vi "calculate.vi"(9 "专项附加扣除（元）":dbl format="%#.3f", 10 "五险一金扣除（元）":dbl format="%#.3f", 11 "年薪金所得（元）":dbl format="%#.3f") -> (0 "抵扣2":dbl, 1 "抵扣1":dbl, 3 "汇算结果（供参考）":string, 4 "税":dbl, 5 "总收入":dbl)   [LabVIEW 2016, in "Tax_calculation.lvclass"]
uses:
  Tax_calculation.lvclass
  <vilib>/Utility/miscctls.llb/LVPointTypeDef.ctl
  PublicSubvi/BoolACT.ctl
  tax list.vi
panel:
  out "reference out":refnum<vi>
  in  "Tab Control":enum32{"综合年度个税汇算", "月度个税计算（预算）"}(tab)
  in  "list":bool
  in  "RESET":bool
  in  "OK":bool
  # "收入"
  # "扣除"
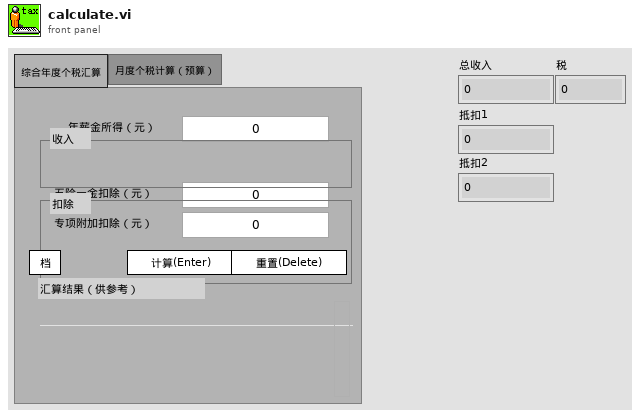
[diagram p1: front panel]
types:
  T1 = typedef "LVPointTypeDef.ctl" = cluster{"Horizontal":i16, "Vertical":i16}
  T2 = cluster{"年薪金所得（元）":refnum<vi>, "五险一金扣除（元）":refnum<vi>, "专项附加扣除（元）":refnum<vi>}
  T3 = enum8{"Enabled", "Disabled", "Disabled and Grayed Out"}
  T4 = typedef "BoolACT.ctl" = enum16{"Get", "Set"}
  T5 = enum32{"Invalid", "Standard", "Closed", "Hidden", "Minimized", "Maximized"}
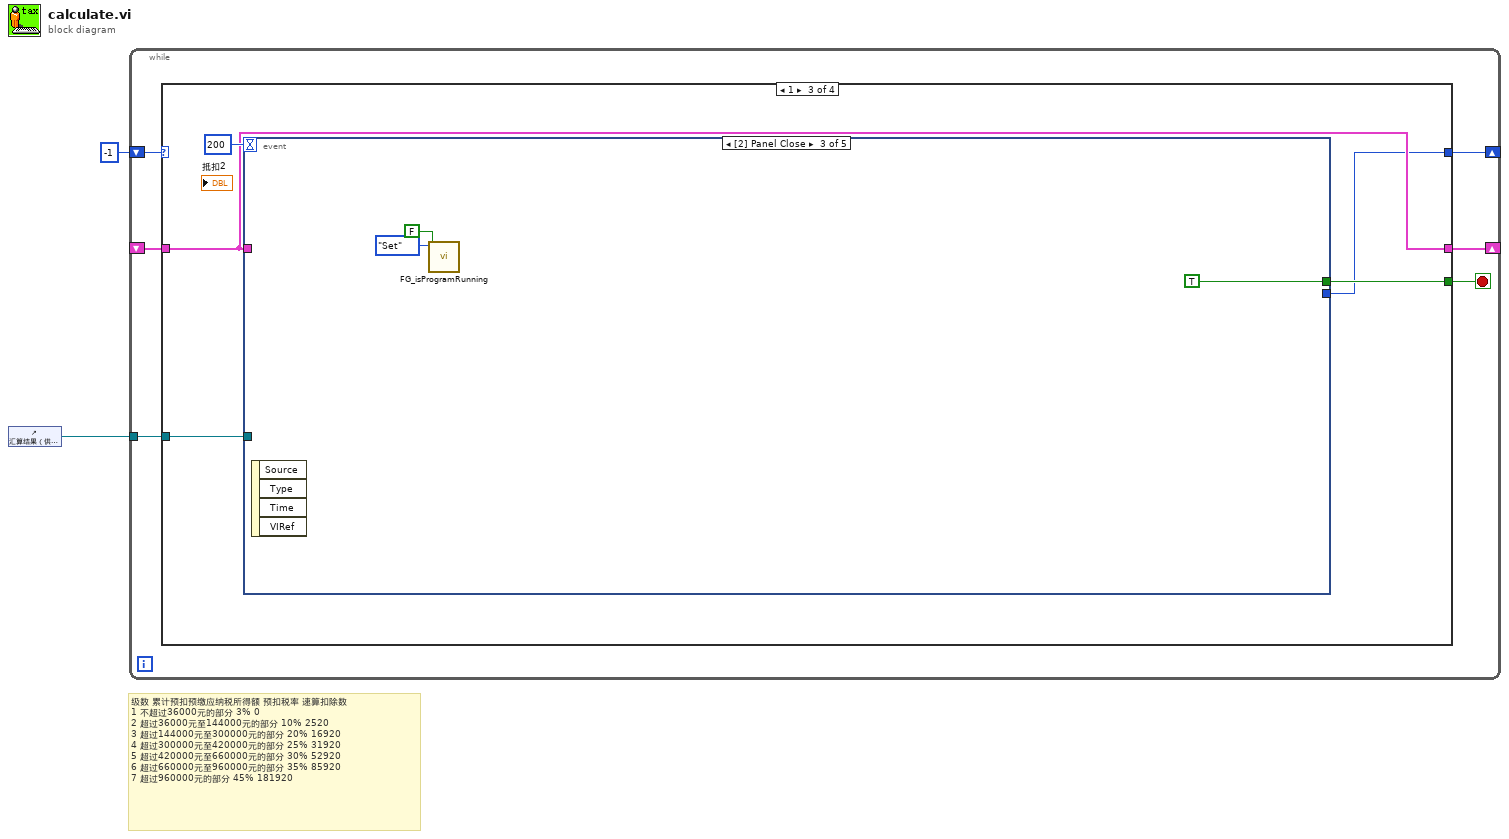
[diagram p0: block diagram]
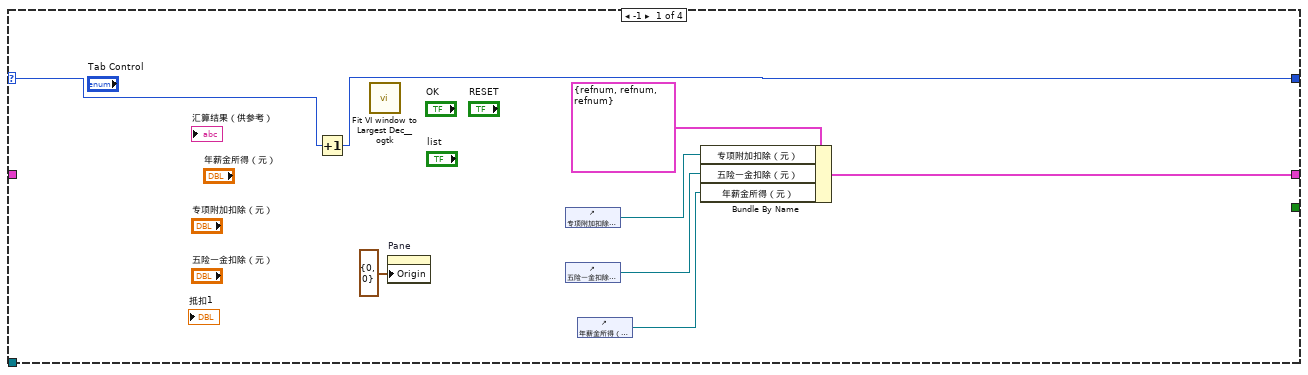
[diagram p2: hidden frame]
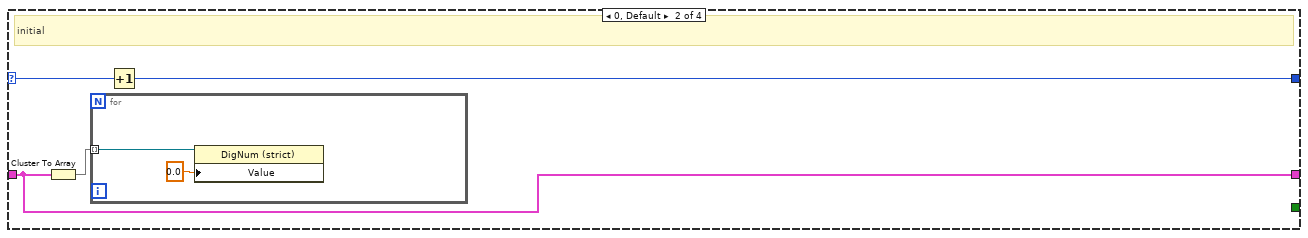
[diagram p3: hidden frame]
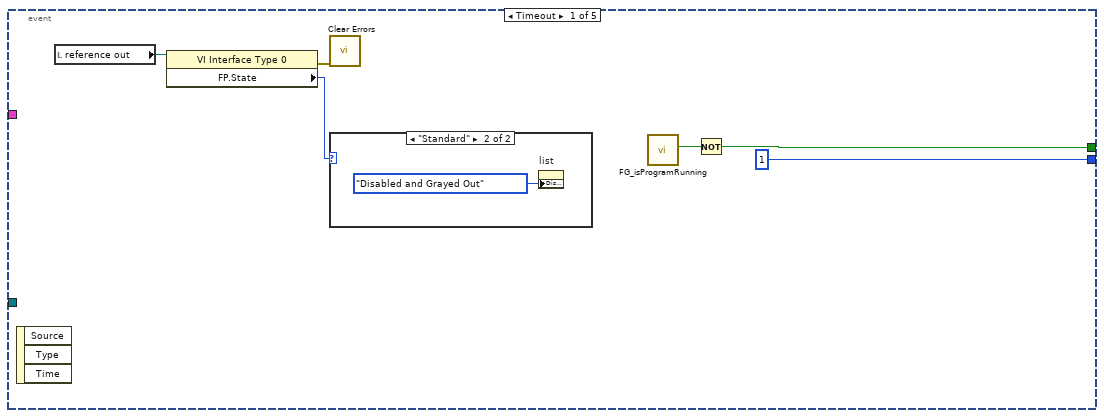
[diagram p4: hidden frame]
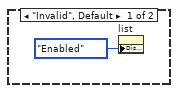
[diagram p5: hidden frame]
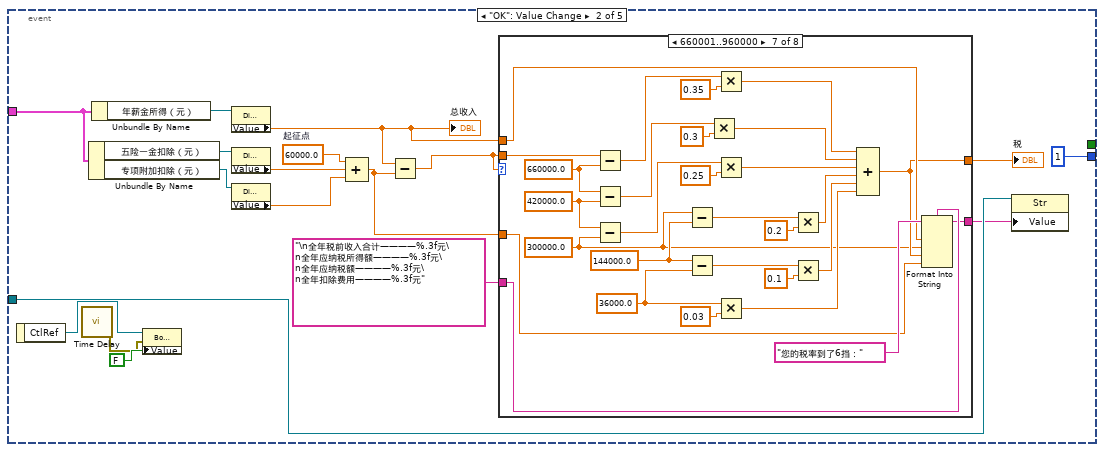
[diagram p6: hidden frame]
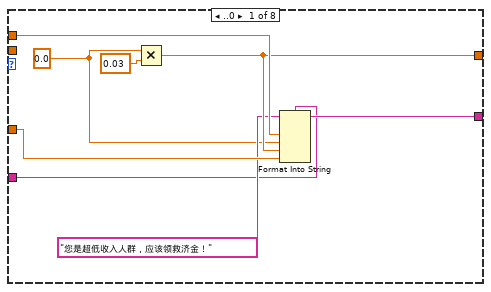
[diagram p7: hidden frame]
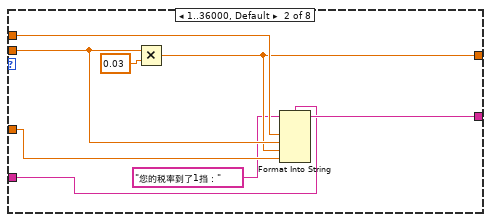
[diagram p8: hidden frame]
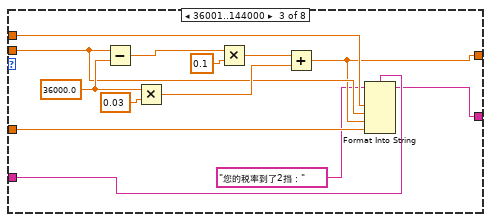
[diagram p9: hidden frame]
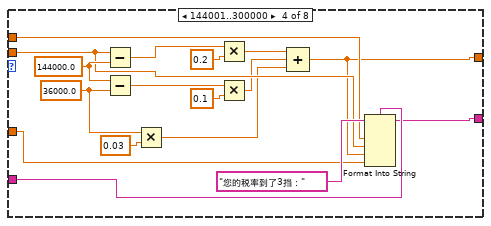
[diagram p10: hidden frame]
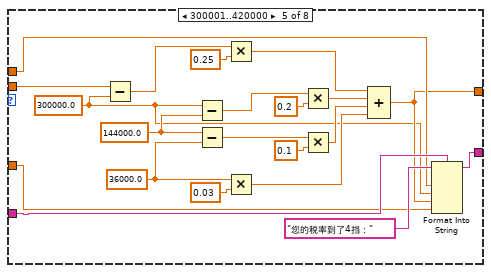
[diagram p11: hidden frame]
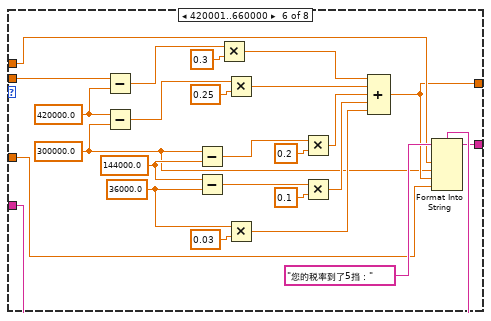
[diagram p12: hidden frame]
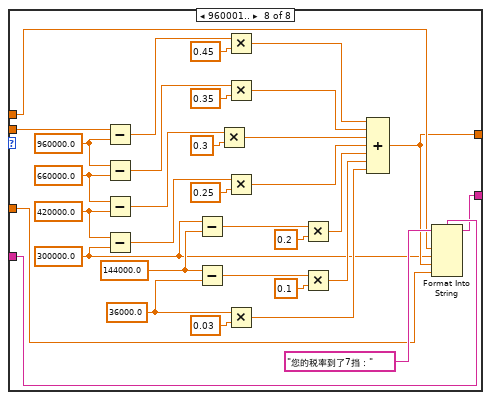
[diagram p13: hidden frame]
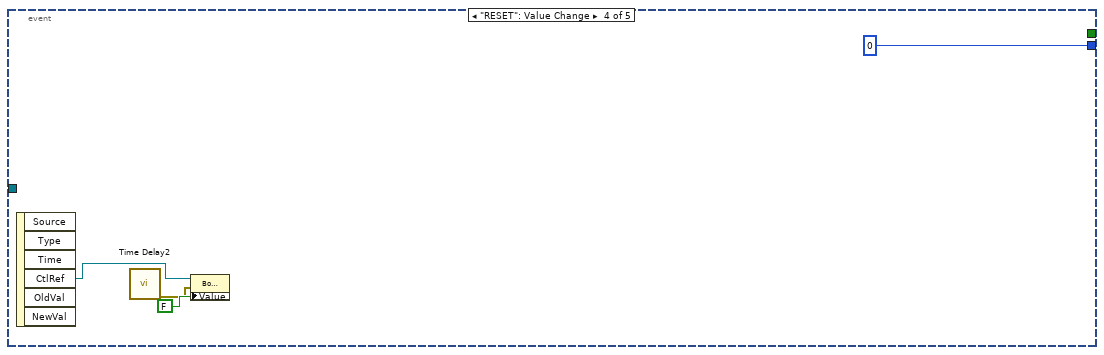
[diagram p14: hidden frame]
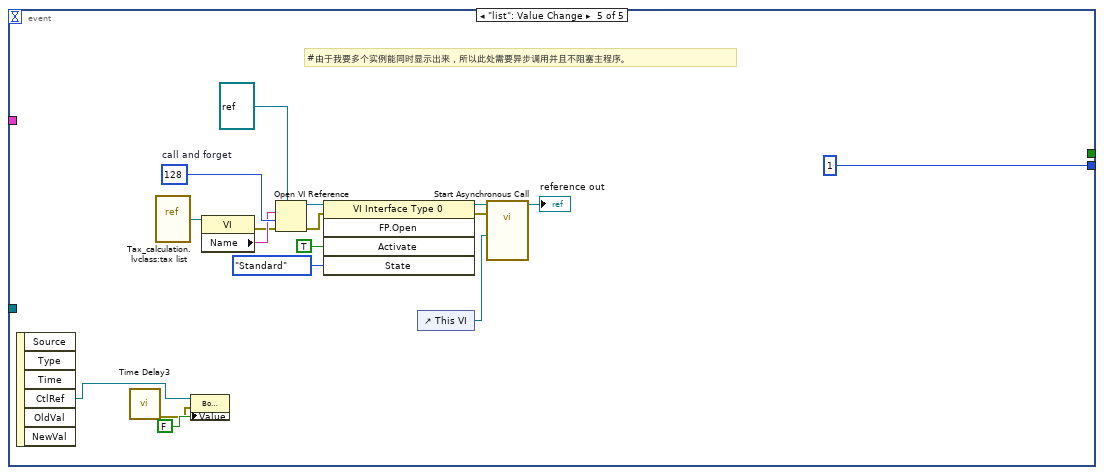
[diagram p15: hidden frame]
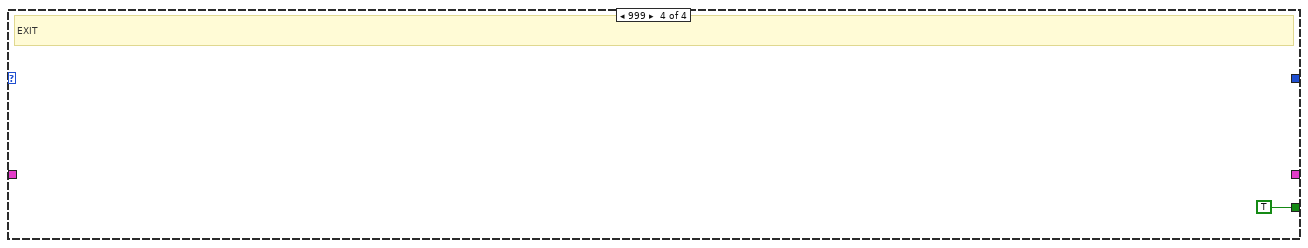
[diagram p16: hidden frame]
diagram:
  # "级数\t累计预扣预缴应纳税所得额\t预扣税率\t速算扣除数\n1\t不超过36000元的部分\t3%\t0\n2\t超过36000元至144000元的部分\t10%\t2520\n3\t超过144000元至300000元的部分\t20%\t16920\n4\t超过300000元至420000元的部分\t25%\t31920\n5\t超过420000元至660000元的部分\t30%\t52920\n6\t超过660000元至960000元的部分\t35%\t85920\n7\t超过960000元的部分\t45%\t181920"
  n1 = control-ref of="汇算结果（供参考）"() -> (w1:refnum<vi>)
  n2 = while {
    shift-right: [w4] -> _
    shift-left: -1 -> [w8]
    shift-right: [w7] -> _
    shift-left: _ -> [w6]
    tunnel: w1 -> [w3]
    stop <- w5 stop-if-true
    n3 = case shown="1" w8 {
      selector: w8 -> [w11 w19 _ _]
      tunnel: [w12 w20 w26 _] -> w7
      tunnel: w6 -> [_ w20 w26 _]
      tunnel: [_ _ w25 TRUE] -> w5
      tunnel: [w10 w18 w23 _] -> w4
      tunnel: w3 -> [_ _ w24 _]
      frame -1 {
        n4 = Increment(x=w11) -> (x+1=w10:i32)
        n5 = call <userlib>:"Fit VI window to Largest Dec__ogtk.vi"() -> ()  [unwired: 6 in, 2 out]
        n6 = property on="Pane" class="Pane"("Origin"=T1 {"Horizontal"=0, "Vertical"=0}) -> ()  [unwired: 2 in, 2 out]
        n7 = control-ref of="专项附加扣除（元）"() -> (w15:refnum<vi>)
        n8 = control-ref of="五险一金扣除（元）"() -> (w14:refnum<vi>)
        n9 = control-ref of="年薪金所得（元）"() -> (w13:refnum<vi>)
        n10 = Bundle By Name(cluster=T2 {"年薪金所得（元）"=refnum, "五险一金扣除（元）"=refnum, "专项附加扣除（元）"=refnum}, "专项附加扣除（元）"=w15, "五险一金扣除（元）"=w14, "年薪金所得（元）"=w13) -> (w12:T2)
      }
      frame 0, Default {
        # "initial"
        n11 = Cluster To Array(cluster=w20) -> (array=w17:refnum<vi>[])
        n12 = for {
          tunnel: w17 -> [w22] mode=indexing
          n13 = property class="DigNum (strict)"(reference=w22, "Value"=0.0) -> ()  [unwired: 1 in, 2 out]
        }
        n14 = Increment(x=w19) -> (x+1=w18:i32)
      }
      frame 1 {
        n15 = event shown="[2] Panel Close" {
          selector: _ -> [_ _ _ _ _]
          dyn-events: _ -> [_ _ _ _ _]
          timeout: 200 -> [_ _ _ _ _]
          tunnel: w26 -> [_ w52 _ _ _]
          tunnel: [w28 _ TRUE _ _] -> w25
          tunnel: w24 -> [_ w47 _ _ _]
          tunnel: [1 1 _ 0 1] -> w23
          event Timeout {
            n16 = event-data() -> ()  [unwired: 1 in, 3 out]
            n17 = local read "reference out"() -> (w33:refnum<vi>)
            n18 = property class="VI Interface Type 0"(reference=w33) -> (error out=w32:errorcluster, "FP.State"=w31:T5)  [unwired: 1 in, 1 out]
            n19 = call <vilib>:"Clear Errors.vi"("error in (no error)"=w32) -> ()  [unwired: 5 in, 2 out]
            n20 = case shown="\"Standard\"" w31 {
              frame "Invalid", Default {
                n21 = property on="list" class="Bool (strict)"("DisabledEnum"=T3."Enabled" ("Disabled")) -> ()  [unwired: 2 in, 2 out]
              }
              frame "Standard" {
                n22 = property on="list" class="Bool (strict)"("DisabledEnum"=T3."Disabled and Grayed Out" ("Disabled")) -> ()  [unwired: 2 in, 2 out]
              }
            }
            n23 = call "FG_isProgramRunning"() -> ("Value"=w29:bool)  [unwired: 10 in, 1 out]
            n24 = Not(x=w29) -> (.not. x?=w28:bool)
          }
          event "OK": Value Change {
            w40 = 60000.0  # 起征点
            n25 = event-data() -> ("CtlRef"=w38:refnum<vi>)  [unwired: 1 in]
            n26 = call "Time Delay"() -> ("error out"=w36:errorcluster)  [unwired: 11 in]
            n27 = Unbundle By Name(w52) -> ("五险一金扣除（元）"=w51:refnum<vi>, "专项附加扣除（元）"=w50:refnum<vi>)
            n28 = Unbundle By Name(w52) -> ("年薪金所得（元）"=w53:refnum<vi>)
            n29 = property class="Bool (strict)"(reference=w38, error in=w36, "Value"=FALSE) -> ()  [unwired: 2 out]
            n30 = property class="DigNum (strict)"(reference=w53) -> ("Value"=w39:dbl)  [unwired: 1 in, 2 out]
            "总收入" <- w39
            n31 = property class="DigNum (strict)"(reference=w51) -> ("Value"=w46:dbl)  [unwired: 1 in, 2 out]
            n32 = property class="DigNum (strict)"(reference=w50) -> ("Value"=w49:dbl)  [unwired: 1 in, 2 out]
            n33 = Compound Arithmetic op=ADD(w40, w46, w49) -> (w44:dbl)
            n34 = Subtract(x=w39, y=w44) -> (x-y=w45:dbl)
            n35 = case shown="660001..960000" w45 {
              tunnel: [w59 w66 w73 w86 w108 w133 w162 w195] -> w48
              tunnel: w45 -> [_ w67 w74 w87 w104 w122 w148 w177]
              tunnel: w39 -> [w60 w68 w75 w88 w109 w134 w163 w196]
              tunnel: w44 -> [w58 w65 w72 w85 w107 w132 w161 w194]
              tunnel: [w57 w64 w70 w90 w111 w136 w165 w198] -> w43
              tunnel: "\n全年税前收入合计————%.3f元\n全年应纳税所得额————%.3f元\n全年应纳税额————%.3f元\n全年扣除费用————%.3f元" ("format string") -> [w55 w62 w76 w91 w112 w137 w166 w199]
              frame ..0 {
                w54 = 0.0
                n36 = Multiply(x=w54, y=0.03) -> (x*y=w59:dbl)
                n37 = Format Into String(format string=w55, initial string="您是超低收入人群，应该领救济金！", w60, w54, w59, w58) -> (resulting string=w57:string)  [unwired: 1 in, 1 out]
              }
              frame 1..36000, Default {
                n38 = Multiply(x=w67, y=0.03) -> (x*y=w66:dbl)
                n39 = Format Into String(format string=w62, initial string="您的税率到了1挡：", w68, w67, w66, w65) -> (resulting string=w64:string)  [unwired: 1 in, 1 out]
              }
              frame 36001..144000 {
                w78 = 36000.0
                n40 = Subtract(x=w74, y=w78) -> (x-y=w82:dbl)
                n41 = Multiply(x=w78, y=0.03) -> (x*y=w77:dbl)
                n42 = Multiply(x=w82, y=0.1) -> (x*y=w81:dbl)
                n43 = Add(x=w81, y=w77) -> (x+y=w73:dbl)
                n44 = Format Into String(format string=w76, initial string="您的税率到了2挡：", w75, w74, w73, w72) -> (resulting string=w70:string)  [unwired: 1 in, 1 out]
              }
              frame 144001..300000 {
                w97 = 144000.0 ("x")
                w92 = 36000.0
                n45 = Subtract(x=w87, y=w97) -> (x-y=w96:dbl)
                n46 = Subtract(x=w97, y=w92) -> (x-y=w93:dbl)
                n47 = Multiply(x=w92, y=0.03) -> (x*y=w83:dbl)
                n48 = Multiply(x=w96, y=0.2) -> (x*y=w94:dbl)
                n49 = Multiply(x=w93, y=0.1) -> (x*y=w84:dbl)
                n50 = Compound Arithmetic op=ADD(w94, w84, w83) -> (w86:dbl)
                n51 = Format Into String(format string=w91, initial string="您的税率到了3挡：", w88, w87, w86, w85) -> (resulting string=w90:string)  [unwired: 1 in, 1 out]
              }
              frame 300001..420000 {
                w100 = 300000.0 ("x")
                w118 = 144000.0 ("x")
                w113 = 36000.0
                n52 = Subtract(x=w104, y=w100) -> (x-y=w102:dbl)
                n53 = Subtract(x=w100, y=w118) -> (x-y=w117:dbl)
                n54 = Subtract(x=w118, y=w113) -> (x-y=w114:dbl)
                n55 = Multiply(x=w102, y=0.25) -> (x*y=w101:dbl)
                n56 = Multiply(x=w113, y=0.03) -> (x*y=w105:dbl)
                n57 = Multiply(x=w117, y=0.2) -> (x*y=w115:dbl)
                n58 = Multiply(x=w114, y=0.1) -> (x*y=w106:dbl)
                n59 = Compound Arithmetic op=ADD(w101, w115, w106, w105) -> (w108:dbl)
                n60 = Format Into String(format string=w112, initial string="您的税率到了4挡：", w109, w100, w108, w107) -> (resulting string=w111:string)  [unwired: 1 in, 1 out]
              }
              frame 420001..660000 {
                w123 = 420000.0 ("x")
                w126 = 300000.0 ("x")
                w143 = 144000.0 ("x")
                w138 = 36000.0
                n61 = Subtract(x=w122, y=w123) -> (x-y=w125:dbl)
                n62 = Subtract(x=w123, y=w126) -> (x-y=w128:dbl)
                n63 = Subtract(x=w126, y=w143) -> (x-y=w142:dbl)
                n64 = Subtract(x=w143, y=w138) -> (x-y=w139:dbl)
                n65 = Multiply(x=w125, y=0.3) -> (x*y=w121:dbl)
                n66 = Multiply(x=w128, y=0.25) -> (x*y=w127:dbl)
                n67 = Multiply(x=w138, y=0.03) -> (x*y=w130:dbl)
                n68 = Multiply(x=w142, y=0.2) -> (x*y=w140:dbl)
                n69 = Multiply(x=w139, y=0.1) -> (x*y=w131:dbl)
                n70 = Compound Arithmetic op=ADD(w121, w127, w140, w131, w130) -> (w133:dbl)
                n71 = Format Into String(format string=w137, initial string="您的税率到了5挡：", w134, w126, w133, w132) -> (resulting string=w136:string)  [unwired: 1 in, 1 out]
              }
              frame 660001..960000 {
                w147 = 660000.0 ("x")
                w152 = 420000.0 ("x")
                w155 = 300000.0 ("x")
                w172 = 144000.0 ("x")
                w167 = 36000.0
                n72 = Subtract(x=w148, y=w147) -> (x-y=w149:dbl)
                n73 = Subtract(x=w147, y=w152) -> (x-y=w154:dbl)
                n74 = Subtract(x=w152, y=w155) -> (x-y=w157:dbl)
                n75 = Subtract(x=w155, y=w172) -> (x-y=w171:dbl)
                n76 = Subtract(x=w172, y=w167) -> (x-y=w168:dbl)
                n77 = Multiply(x=w154, y=0.3) -> (x*y=w151:dbl)
                n78 = Multiply(x=w149, y=0.35) -> (x*y=w146:dbl)
                n79 = Multiply(x=w157, y=0.25) -> (x*y=w156:dbl)
                n80 = Multiply(x=w167, y=0.03) -> (x*y=w159:dbl)
                n81 = Multiply(x=w171, y=0.2) -> (x*y=w169:dbl)
                n82 = Multiply(x=w168, y=0.1) -> (x*y=w160:dbl)
                n83 = Compound Arithmetic op=ADD(w146, w151, w156, w169, w160, w159) -> (w162:dbl)
                n84 = Format Into String(format string=w166, initial string="您的税率到了6挡：", w163, w155, w162, w161) -> (resulting string=w165:string)  [unwired: 1 in, 1 out]
              }
              frame 960001.. {
                w176 = 960000.0 ("x")
                w181 = 660000.0 ("x")
                w185 = 420000.0 ("x")
                w188 = 300000.0 ("x")
                w205 = 144000.0 ("x")
                w200 = 36000.0
                n85 = Subtract(x=w177, y=w176) -> (x-y=w179:dbl)
                n86 = Subtract(x=w176, y=w181) -> (x-y=w182:dbl)
                n87 = Subtract(x=w181, y=w185) -> (x-y=w187:dbl)
                n88 = Subtract(x=w185, y=w188) -> (x-y=w190:dbl)
                n89 = Subtract(x=w188, y=w205) -> (x-y=w204:dbl)
                n90 = Subtract(x=w205, y=w200) -> (x-y=w201:dbl)
                n91 = Multiply(x=w187, y=0.3) -> (x*y=w184:dbl)
                n92 = Multiply(x=w179, y=0.45) -> (x*y=w175:dbl)
                n93 = Multiply(x=w182, y=0.35) -> (x*y=w180:dbl)
                n94 = Multiply(x=w190, y=0.25) -> (x*y=w189:dbl)
                n95 = Multiply(x=w200, y=0.03) -> (x*y=w192:dbl)
                n96 = Multiply(x=w204, y=0.2) -> (x*y=w202:dbl)
                n97 = Multiply(x=w201, y=0.1) -> (x*y=w193:dbl)
                n98 = Compound Arithmetic op=ADD(w175, w180, w184, w189, w202, w193, w192) -> (w195:dbl)
                n99 = Format Into String(format string=w199, initial string="您的税率到了7挡：", w196, w188, w195, w194) -> (resulting string=w198:string)  [unwired: 1 in, 1 out]
              }
            }
            "税" <- w48
            n100 = property class="Str"(reference=w47, "Value"=w43) -> ()  [unwired: 1 in, 2 out]
          }
          event Panel Close {
            n101 = event-data() -> ()  [unwired: 1 in, 4 out]
            n102 = call "FG_isProgramRunning"("Value"=FALSE, "ACT"=BoolACT."Set") -> ()  [unwired: 8 in, 2 out]
          }
          event "RESET": Value Change {
            n103 = event-data() -> ("CtlRef"=w211:refnum<vi>)  [unwired: 1 in, 5 out]
            n104 = call "Time Delay2"() -> ("error out"=w212:errorcluster)  [unwired: 11 in]
            n105 = property class="Bool (strict)"(reference=w211, error in=w212, "Value"=FALSE) -> ()  [unwired: 2 out]
          }
          event "list": Value Change {
            w225 = 128  # call and forget
            # "#由于我要多个实例能同时显示出来，所以此处需要异步调用并且不阻塞主程序。"
            n106 = event-data() -> ("CtlRef"=w228:refnum<vi>)  [unwired: 1 in, 5 out]
            n107 = call "Time Delay3"() -> ("error out"=w229:errorcluster)  [unwired: 11 in]
            n108 = vi-ref "Tax_calculation.lvclass:tax list.vi"() -> (w221:refnum<vi>)
            n109 = property class="Bool (strict)"(reference=w228, error in=w229, "Value"=FALSE) -> ()  [unwired: 2 out]
            n110 = property class="VI"(reference=w221) -> (error out=w222:errorcluster, "Name"=w223:string)  [unwired: 1 in, 1 out]
            n111 = Open VI Reference(type specifier VI Refnum (for type only)=refnum<vi> refnum, vi path=w223, options=w225, error in (no error)=w222) -> (vi reference=w220:refnum<vi>, error out=w218:errorcluster)  [unwired: 2 in]
            n112 = invoke class="VI Interface Type 0" method="FP.Open"(reference=w220, error in=w218, "Activate"=TRUE ("Activate?"), "State"=T5."Standard") -> (reference out=w219:refnum<vi>, error out=w217:errorcluster)  [unwired: 1 in, 3 out]
            n113 = control-ref of="This VI"() -> (w216:refnum<vi>)
            n114 = call-by-ref "Start Asynchronous Call"(reference=w219, error in=w217, "Parren VI"=w216) -> (reference out=→"reference out":refnum<vi>)  [unwired: 11 in, 1 out]
          }
        }
      }
      frame 999 {
        # "EXIT"
      }
    }
  }
